vi "WriteFailCount.vi"(7 "SequenceFillePath":string, 8 "error in (no error)":errorcluster, 9 "Fail":u32, 10 "Pass":u32, 11 "Statistics path":path) -> (0 "error out":errorcluster, 3 "file path":path)   [LabVIEW 2019, in "TestBench.lvlib" / "TestBench.lvclass"]
uses:
  TestBench.lvclass
  <vilib>/Utility/config.llb/Write Key (U32).vi
  <vilib>/Utility/config.llb/NI_LVConfig.lvlib
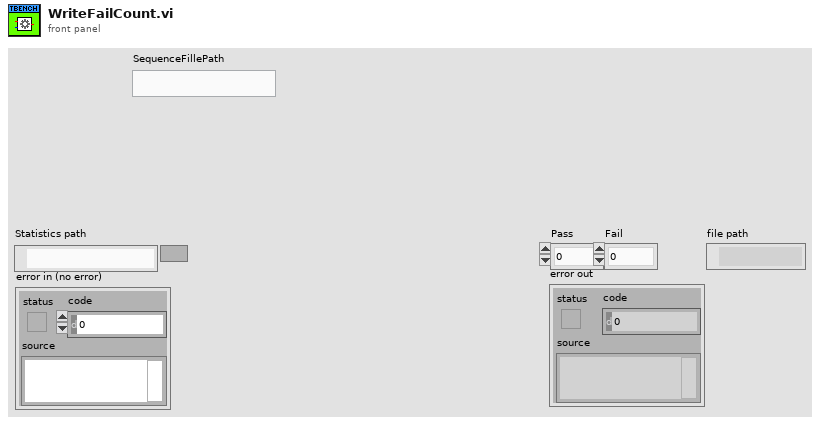
[diagram p1: front panel]
types:
  T1 = typedef "NI_LVConfig.lvlib/Config Data RefNum.ctl" = refnum<k1>
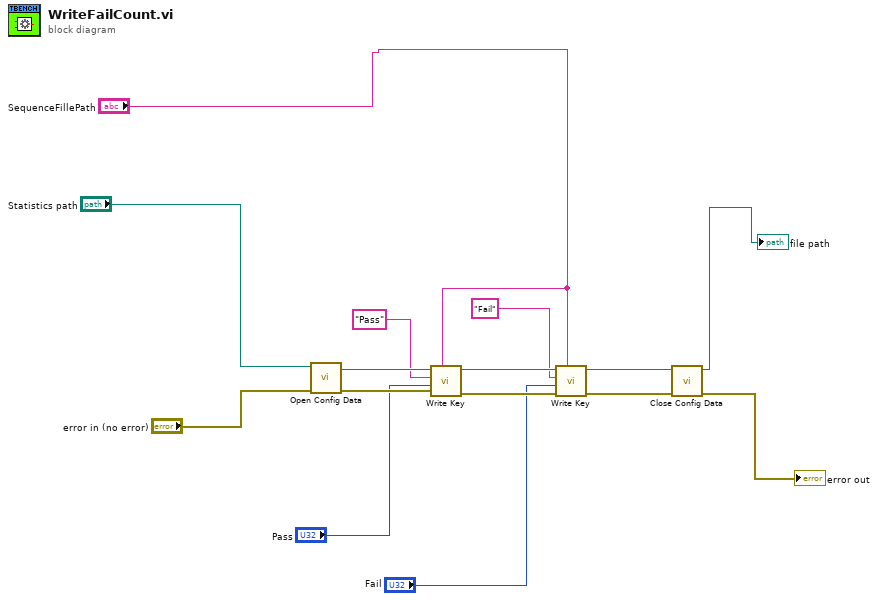
[diagram p0: block diagram]
diagram:
  n1 = call <vilib>:"Open Config Data.vi"("error in (no error)"="error in (no error)", "configuration file path"="Statistics path") -> ("error out"=w13:errorcluster, "refnum"=w14:T1)  [unwired: 7 in, 1 out]
  n2 = call-poly <vilib>:"Write Key.vi"("section"="SequenceFillePath", "error in (no error)"=w13, "value"="Pass", "key"="Pass", "refnum"=w14) -> ("error out"=w10:errorcluster, "refnum out"=w11:T1)  [unwired: 4 in, 1 out]
  n3 = call-poly <vilib>:"Write Key.vi"("section"="SequenceFillePath", "error in (no error)"=w10, "value"="Fail", "key"="Fail", "refnum"=w11) -> ("error out"=w7:errorcluster, "refnum out"=w8:T1)  [unwired: 4 in, 1 out]
  n4 = call <vilib>:"Close Config Data.vi"("error in (no error)"=w7, "refnum"=w8) -> ("error out"=→"error out":errorcluster, "file path"=→"file path":path)  [unwired: 8 in]
